vi "Start USB Default.vi"(0 "Device ID":T1(ring), 2 "Distance Sensor Mode":enum32{"Voltage", "Distance"}(ring)=enum."Distance", 11 "error in":errorcluster) -> (4 "Device ID Out":T1(ring), 15 "error out":errorcluster)   [LabVIEW 2010]
doc: "This VI is for the Robo Interface Only - This VI opens USB communication between your computer and the Robo Interface. Then, it uses default settings to configure the digital distance sensors. Last, it starts the transfer area which is where the Robo Interface writes data to be read and reads data to be written."
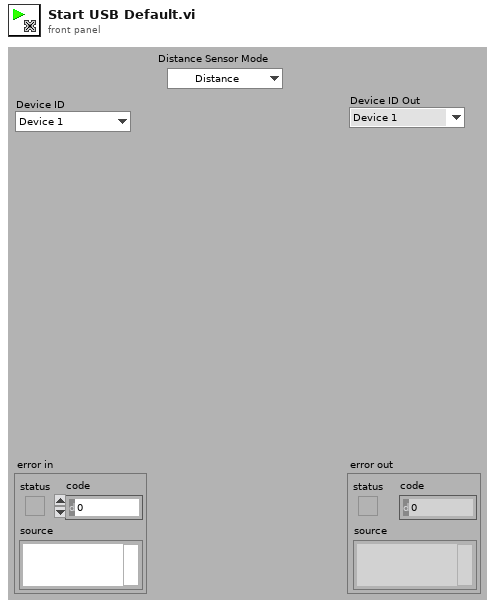
[diagram p1: front panel]
types:
  T1 = enum16{"Device 1", "Device 2", "Device 3", "Device 4", "Device 5", "Device 6", "Device 7", "Device 8"}
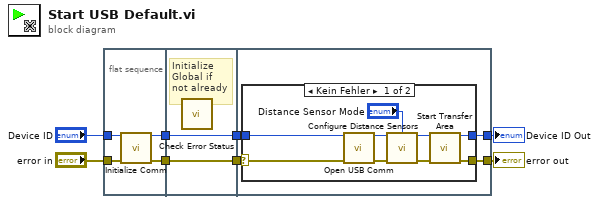
[diagram p0: block diagram]
diagram:
  n1 = flat-sequence {
    tunnel: "error in" -> [w10]
    tunnel: "Device ID" -> [w12]
    tunnel: [w11] -> w2
    tunnel: [w9] -> w1
    tunnel: [w14] -> w7
    tunnel: [w13] -> w6
    tunnel: w2 -> [w14]
    tunnel: w1 -> [w13]
    tunnel: w7 -> [w18]
    tunnel: w6 -> [w17]
    tunnel: [w16] -> w4
    tunnel: [w15] -> w3
    frame #0 {
      n2 = call "Initialize Comm.vi"("Device ID"=w12, "error in"=w10) -> ("Device ID Out"=w11:T1, "error out"=w9:errorcluster)  [unwired: 1 in, 11 out]
    }
    frame #1 {
      # "Initialize\nGlobal if\nnot already"
      n3 = call "Check Error Status.vi"() -> ()  [unwired: 3 in, 13 out]
    }
    frame #2 {
      n4 = case shown="Kein Fehler" w17 {
        selector: w17 -> [w23 w29]
        tunnel: [w27 w29] -> w16
        tunnel: w18 -> [w21 w28]
        tunnel: [w26 w28] -> w15
        frame No Error {
          n5 = call "Open USB Comm.vi"("Device ID"=w21, "error in"=w23) -> ("Device ID Out"=w20:T1, "error out"=w22:errorcluster)  [unwired: 12 out]
          n6 = call "Configure Distance Sensors.vi"("Device ID"=w20, "Distance Sensor Mode"="Distance Sensor Mode", "error in"=w22) -> ("Device ID Out"=w24:T1, "error out"=w25:errorcluster)  [unwired: 6 in, 5 out]
          n7 = call "Start Transfer Area.vi"("Device ID"=w24, "error in"=w25) -> ("Device ID Out"=w26:T1, "error out"=w27:errorcluster)  [unwired: 12 out]
        }
        frame Error {
        }
      }
    }
  }
  "error out" <- w4
  "Device ID Out" <- w3
